vi "Start Task.vi"(8 "error in":errorcluster, 10 "Task Ident":string, 11 "Series Actor in":refnum<class "Series Actor.lvclass">) -> (0 "error out":errorcluster, 3 "Series Actor out":refnum<class "Series Actor.lvclass">)   [LabVIEW 2023, in "Series Actor.lvlib" / "Series Actor.lvclass"]
uses:
  Series Actor.lvclass
  Series Actor.lvclass/Series Actor.ctl
  <vilib>/ActorFramework/Message Enqueuer/Message Enqueuer.lvclass/Message Enqueuer.ctl
  <vilib>/ActorFramework/Message Enqueuer/Enqueue.vi
  Task/ITask Actor/ITask Actor Messages/Start Msg/Start Msg.lvclass
  <vilib>/Utility/LVClass/Get LV Class Name.vi
  <resource>/AFDebug/Generate Trace for Message.vi
  <vilib>/ActorFramework/Message Priority Queue/Priority Enqueue.vi
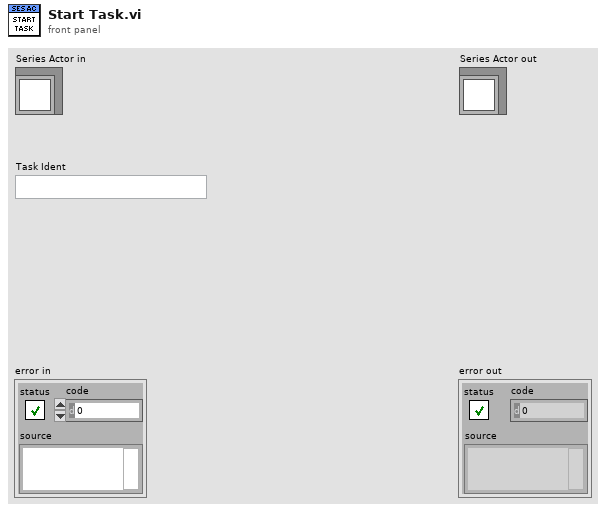
[diagram p1: front panel]
types:
  T1 = map{string, refnum<class "Message Enqueuer.lvclass">}
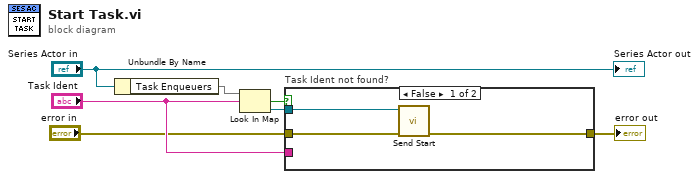
[diagram p0: block diagram]
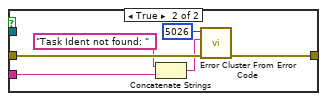
[diagram p2: hidden frame]
diagram:
  n1 = Unbundle By Name("Series Actor in") -> ("Task Enqueuers"=w3:T1)
  n2 = Look In Map(map=w3, key="Task Ident") -> (key not found?=w2:bool, value=w1:refnum<class "Message Enqueuer.lvclass">)  [unwired: 1 in]
  n3 = case "Task Ident not found?" shown="False" w2 {
    tunnel: [w10 w11] -> w7
    tunnel: "error in" -> [w9 w16]
    tunnel: w1 -> [w8 _]
    tunnel: "Task Ident" -> [_ w13]
    frame False {
      n4 = call "Send Start.vi"("error in (no error)"=w9, "Message Enqueuer"=w8) -> ("error out"=w10:errorcluster)  [unwired: 8 in, 1 out]
    }
    frame True {
      n5 = Concatenate Strings("Task Ident not found: " ("string"), w13) -> (w14:string)
      n6 = call <vilib>:"Error Cluster From Error Code.vi"("error in (no error)"=w16, "error message (\"\")"=w14, "error code (0)"=5026) -> ("error out"=w11:errorcluster)  [unwired: 6 in]
    }
  }
  "error out" <- w7
  "Series Actor out" <- "Series Actor in"
